vi "Servo_enable.vi"(8 "error in":errorcluster, 9 "Enable 2":bool=TRUE, 10 "Enable":bool=TRUE) -> (0 "error out":errorcluster)   [LabVIEW 2009, in "Servo.lvlib"]
uses:
  Servo.lvlib
  PWM/PWM_Name.ctl
  PWM.lvlib
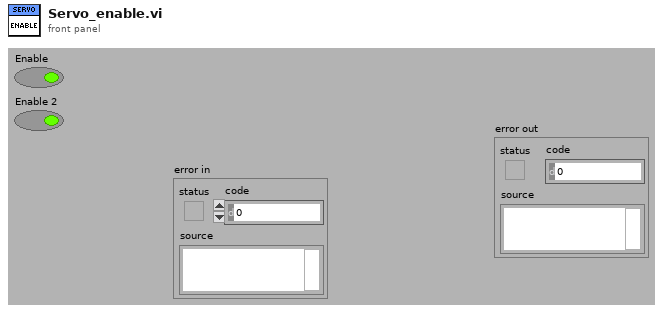
[diagram p1: front panel]
types:
  T1 = typedef "PWM.lvlib/PWM_Name.ctl" = u16
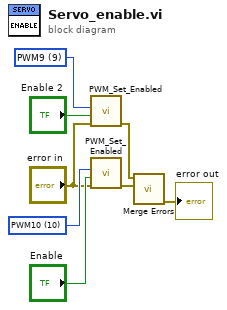
[diagram p0: block diagram]
diagram:
  w4 = T1 10 items=["Invalid"=0, "PWM1"=1, "PWM2"=2, "PWM9"=9, "PWM10"=10] ("PWM_in")
  w5 = T1 9 items=["Invalid"=0, "PWM1"=1, "PWM2"=2, "PWM9"=9, "PWM10"=10] ("PWM_in")
  n1 = call "PWM_Set_Enabled.vi"("error in"="error in", "Enable"="Enable 2", "PWM_in"=w5) -> ("error out"=w7:errorcluster)  [unwired: 7 in, 1 out]
  n2 = call "PWM_Set_Enabled.vi"("error in"="error in", "Enable"="Enable", "PWM_in"=w4) -> ("error out"=w6:errorcluster)  [unwired: 7 in, 1 out]
  n3 = call <vilib>:"Merge Errors.vi"("error in 2 (no error)"=w6, "error in 1 (no error)"=w7) -> ("error out"=→"error out":errorcluster)  [unwired: 5 in]
